vi "Construct Root Model Publishes Double Float.vi"(10 "Datum Name":string) -> (1 "Error Notifier":refnum<notifier>, 3 "RootModelPublishesDoubleFloat out":refnum<class "RootModelPublishesDoubleFloat.lvclass">)   [LabVIEW 2017, in "RootModelPublishesDoubleFloat.lvlib" / "RootModelPublishesDoubleFloat.lvclass"]
uses:
  RootModelPublishesDoubleFloat.lvclass
  RootModelPublishesDoubleFloat.lvclass/RootModelPublishesDoubleFloat.ctl
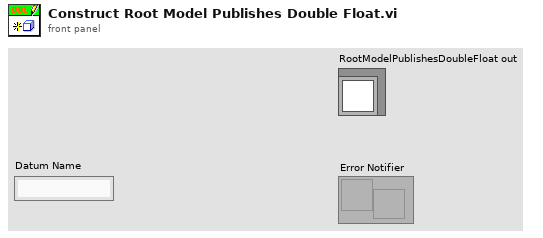
[diagram p1: front panel]
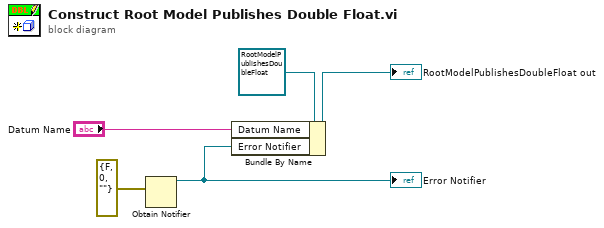
[diagram p0: block diagram]
diagram:
  n1 = Obtain Notifier(notification data type=errorcluster {"status"=FALSE, "code"=0, "source"=""} ("error constant")) -> (notifier out=w1:refnum<notifier>)  [unwired: 3 in, 2 out]
  "Error Notifier" <- w1
  n2 = Bundle By Name(cluster=refnum<class "RootModelPublishesDoubleFloat.lvclass"> refnum ("RootModelPublishesDoubleFloat in"), "Datum Name"="Datum Name", "Error Notifier"=w1) -> (→"RootModelPublishesDoubleFloat out":refnum<class "RootModelPublishesDoubleFloat.lvclass">)
